vi "_075.vi"() -> ()   [LabVIEW 2024]
panel:
  out "deleted portion 1":i32[](array[numeric])
  out "array w/ subset deleted 1":i32[](array[numeric])
  out "deleted portion 2":i32[](array[numeric])
  out "array w/ subset deleted 2":i32[](array[numeric])
  # "Fundamentals :"
  # "4~>After running this VI,what is the value displayed in the o/p ?"
  # "Nrml Approach :"
  # "Dfrnt Approach :"
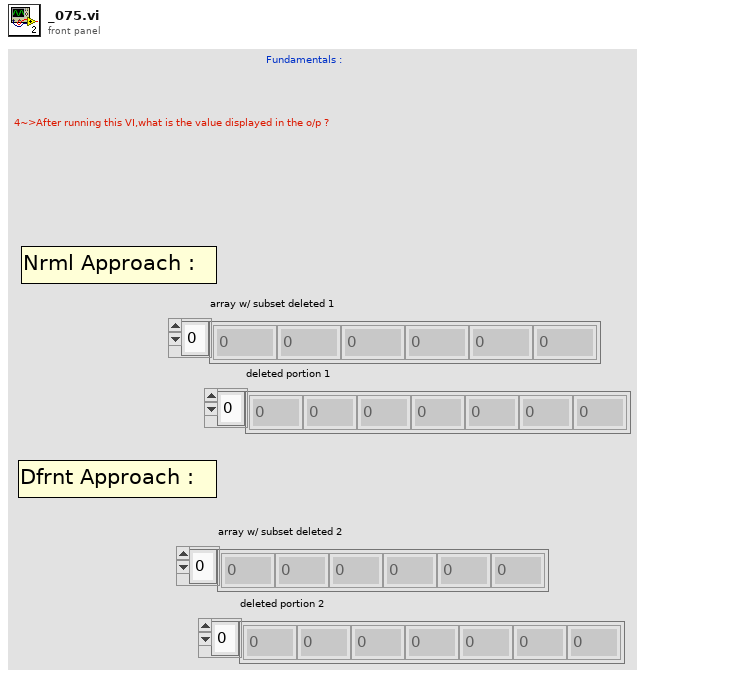
[diagram p1: front panel]
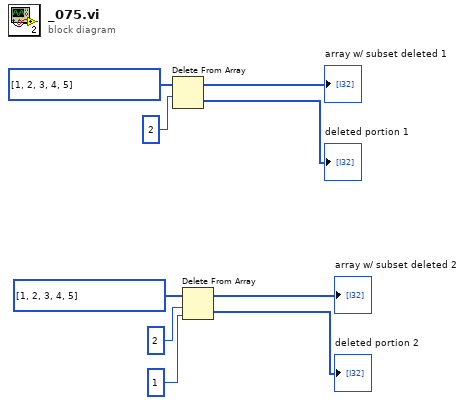
[diagram p0: block diagram]
diagram:
  n1 = Delete From Array "Delete From Array"(array=i32[] [1, 2, 3, 4, 5], length=2) -> (deleted portion=→"deleted portion 1":i32[], array with subset deleted=→"array w/ subset deleted 1":i32[])  [unwired: 1 in]
  n2 = Delete From Array "Delete From Array"(array=i32[] [1, 2, 3, 4, 5], length=2, index=1) -> (deleted portion=→"deleted portion 2":i32[], array with subset deleted=→"array w/ subset deleted 2":i32[])
